vi "Parse Integer String As Quad.vi"(8 "error in (no error)":errorcluster, 10 "Negative":bool, 11 "String":string) -> (0 "error out":errorcluster, 3 "Value":variant)   [LabVIEW 2019, in "JKI JSON Serialization.lvlib" / "JSON Parser.lvclass"]
doc: "JKI JSON 1.1.10.37\nTomi Maila - JKI\nCopyright (c) 2017, JKI"
uses:
  JSON Parser.lvclass
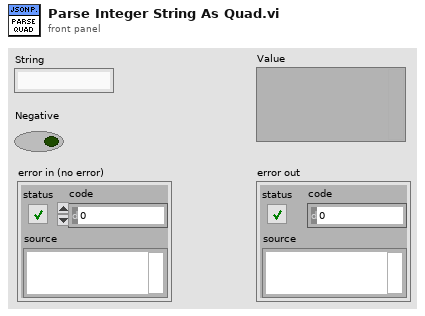
[diagram p1: front panel]
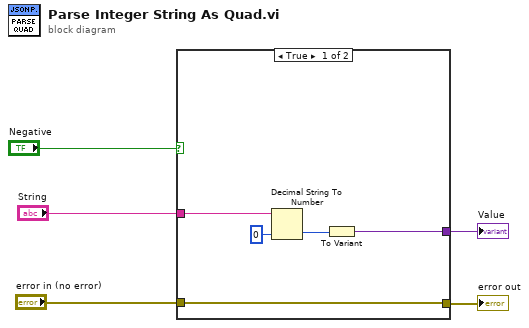
[diagram p0: block diagram]
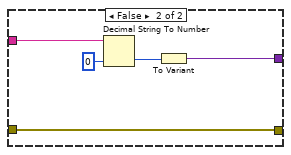
[diagram p2: hidden frame]
diagram:
  n1 = case shown="True" "Negative" {
    tunnel: "String" -> [w10 w15]
    tunnel: [w7 w12] -> w4
    tunnel: "error in (no error)" -> [w6 w11]
    tunnel: [w6 w11] -> w3
    frame True {
      n2 = Decimal String To Number(string=w10, default (0L)=i64 0 ("default (0 I32)")) -> (number=w8:i64)  [unwired: 1 in, 1 out]
      n3 = To Variant(anything=w8) -> (Variant=w7:variant)
    }
    frame False {
      n4 = Decimal String To Number(string=w15, default (0L)=u64 0 ("default (0 I32)")) -> (number=w13:u64)  [unwired: 1 in, 1 out]
      n5 = To Variant(anything=w13) -> (Variant=w12:variant)
    }
  }
  "Value" <- w4
  "error out" <- w3
